vi "_PC_Pub_FM init.vi"(8 "error in (no error)":errorcluster, 11 "FM in":refnum<class "FM.lvclass">) -> (0 "error out":errorcluster, 3 "FM out":refnum<class "FM.lvclass">)   [LabVIEW 2018, in "FM.lvclass"]
uses:
  FM.lvclass
  TDMSAdv.lvclass
  FM.lvclass/FM.ctl
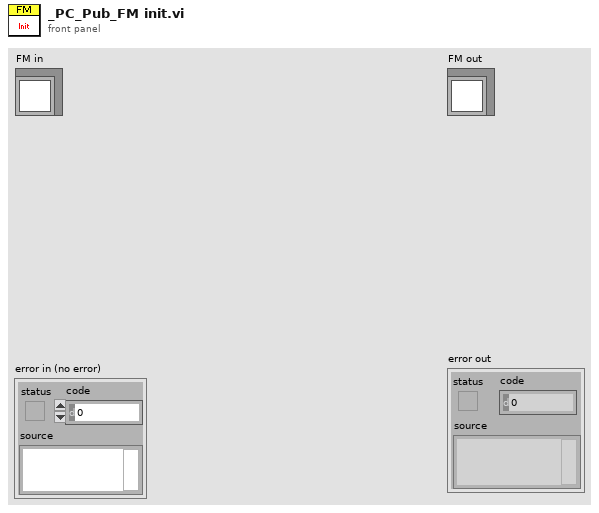
[diagram p1: front panel]
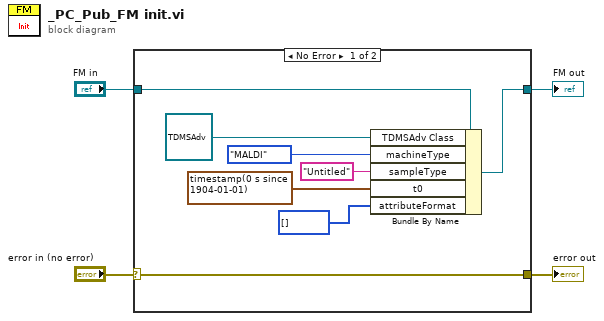
[diagram p0: block diagram]
diagram:
  n1 = case shown="No Error" "error in (no error)" {
    selector: "error in (no error)" -> [w9 w14]
    tunnel: [w9 w14] -> w3
    tunnel: [w12 w13] -> w1
    tunnel: "FM in" -> [w11 w13]
    frame No Error {
      n2 = Bundle By Name(cluster=w11, "TDMSAdv Class"=refnum<class "TDMSAdv.lvclass"> refnum, "machineType"=enum16{"MALDI", "ESI"}."MALDI", "sampleType"="Untitled", "t0"=timestamp(0 s since 1904-01-01), "attributeFormat"=i16[] [] ("AttributeFormat")) -> (w12:refnum<class "FM.lvclass">)
    }
    frame Error {
    }
  }
  "error out" <- w3
  "FM out" <- w1
